vi "MOVE BIAS.vi"(0 "Dx, Dy":cluster{"Dx":sgl, "Dy":sgl}={"Dx"=1e-10, "Dy"=1e-10}, 5 "Initial X":sgl, 7 "Boolean":bool, 9 "Initial Y":sgl) -> (6 "FInal X (m)":sgl, 10 "Final Y (m)":sgl)   [LabVIEW 2025]
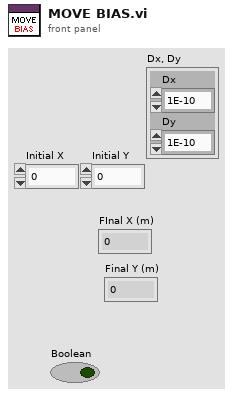
[diagram p1: front panel]
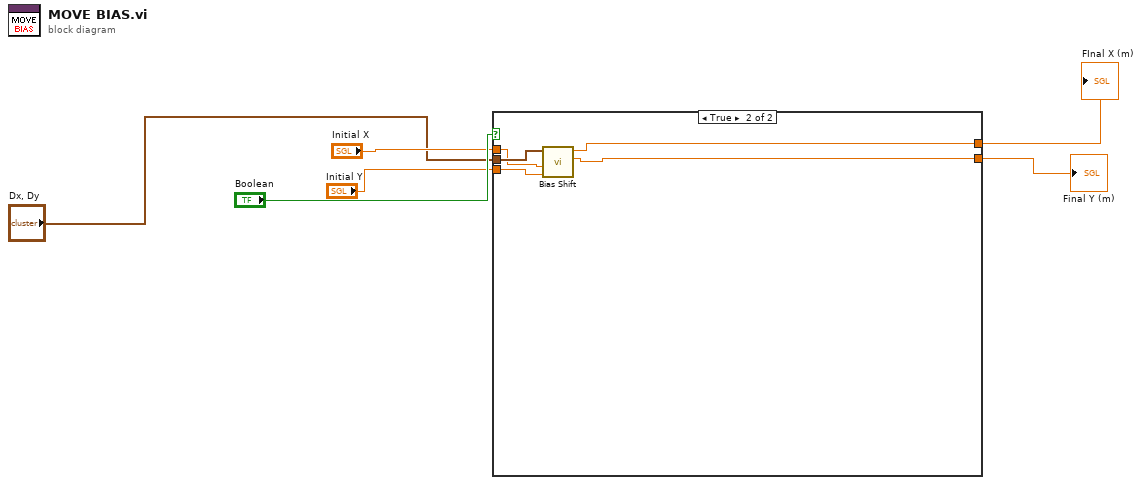
[diagram p0: block diagram]
diagram:
  n1 = case shown="True" "Boolean" {
    tunnel: "Dx, Dy" -> [_ w9]
    tunnel: [_ w11] -> w2
    tunnel: "Initial X" -> [_ w7]
    tunnel: "Initial Y" -> [_ w8]
    tunnel: [_ w10] -> w3
    frame False {
    }
    frame True {
      n2 = call "Bias Shift.vi"("y"=w8, "x"=w7, "Dx, Dy"=w9) -> ("Y (m)"=w10:sgl, "X (m)"=w11:sgl)  [unwired: 7 in]
    }
  }
  "Final Y (m)" <- w3
  "FInal X (m)" <- w2
